vi "I(V)_MFLI_PK_v4.0_measure X.vi"() -> ()   [LabVIEW 2016]
uses:
  Labview Drivers/MFLI/LabOneLabVIEW-22.02.26577/LabOneLabVIEW-22.02.26577/Zurich Instruments LabOne/Public/Data/ziTypeDemodSampleSingle.ctl
  Labview Drivers/MFLI/LabOneLabVIEW-22.02.26577/LabOneLabVIEW-22.02.26577/Zurich Instruments LabOne/Public/Configure/ziSetValueDouble.vi
  Labview Drivers/MFLI/LabOneLabVIEW-22.02.26577/LabOneLabVIEW-22.02.26577/Zurich Instruments LabOne/Public/Configure/ziGetValueDemodSampleEx.vi
  Labview Drivers/MFLI/LabOneLabVIEW-22.02.26577/LabOneLabVIEW-22.02.26577/Zurich Instruments LabOne/Zurich Instruments LabOne.lvlib
panel:
  in  "MFLI Average":i32=1
  out "Resistance (ohm)":dbl=10.271037379735393 format="%#_13g"
  out "R vs V":cluster{dbl, "Field Reading":dbl}[](graph)=[{8.807116465394836e-09, "Field Reading"=-5977.19453137507}, {7.862385412624124e-09, "Field Reading"=0.816626175267259}, {1.016246783678571e-08, "Field Reading"=0.22593081706163012}, {2.8394518144070844e-08, "Field Reading"=0.3244930369790309}, {4.55394808090395e-08, "Field Reading"=0.3437719763523952}, {6.89280912729516e-08, "Field Reading"=0.38589888456590915}, {8.892988920666698e-08, "Field Reading"=0.07130629996454171}, {1.1092974614674399e-07, "Field Reading"=0.2348376343368235}, {1.291523087387538e-07, "Field Reading"=0.37898620517760767}, {1.4722365790221026e-07, "Field Reading"=0.4039183683262634}, {1.807306492808588e-07, "Field Reading"=0.44321715885434587}, {1.9469830782225016e-07, "Field Reading"=0.4299026538647131}, {2.1455394499138842e-07, "Field Reading"=0.43043853663662857}, {2.3655611150765593e-07, "Field Reading"=0.43467611037569903}, {2.59606088721133e-07, "Field Reading"=0.43952372149878877}, {2.758303395650899e-07, "Field Reading"=0.43362275822843394}, {2.898255168785462e-07, "Field Reading"=0.42491475414262025}, {3.1095121503066903e-07, "Field Reading"=0.4281996541380056}, {3.290239859654633e-07, "Field Reading"=0.426217192462996}, {3.440405349336837e-07, "Field Reading"=0.42103190972467763}, {3.67176584323379e-07, "Field Reading"=0.42612243564533486}, {3.8988760409248366e-07, "Field Reading"=0.42973279263530023}, {4.033185654384404e-07, "Field Reading"=0.4229755766582419}, {4.251248472726496e-07, "Field Reading"=0.42533821159897195}, {4.5031688342256917e-07, "Field Reading"=0.43082327628658923}, {4.6749835720727547e-07, "Field Reading"=0.4285130615827359}, {4.868781675265887e-07, "Field Reading"=0.42843576289196017}, {5.115536329406834e-07, "Field Reading"=0.43266001598448733}, {5.343117600631355e-07, "Field Reading"=0.4353606504326838}, {5.541237064759493e-07, "Field Reading"=0.43555248194144336}, {5.726324607401028e-07, "Field Reading"=0.4346915313695261}, {5.873127708721604e-07, "Field Reading"=0.4307903324089991}, {6.019024857908083e-07, "Field Reading"=0.4272258139653861}, {6.223909508091271e-07, "Field Reading"=0.4278930599741731}, {6.425541697267918e-07, "Field Reading"=0.42851691356665206}, {6.687384309745611e-07, "Field Reading"=0.4327338077376769}, {6.88227751334839e-07, "Field Reading"=0.43265173136675905}, {7.032166146053452e-07, "Field Reading"=0.42977933132645724}, {7.224516085197258e-07, "Field Reading"=0.4295413108829304}, {7.474914126034483e-07, "Field Reading"=0.4326650258503734}, {7.733169248070552e-07, "Field Reading"=0.4361152915047444}, {7.885708893571228e-07, "Field Reading"=0.43367432747768353}, {8.069399471456721e-07, "Field Reading"=0.4330162152944697}, {8.337333568827311e-07, "Field Reading"=0.4367253360501215}, {8.502533827097552e-07, "Field Reading"=0.4347849286054917}, {8.646622700555259e-07, "Field Reading"=0.43205649752211134}, {8.808103063521348e-07, "Field Reading"=0.43032588911090636}, {9.07332307666703e-07, "Field Reading"=0.43368905642592026}, {9.20609541766958e-07, "Field Reading"=0.43064678759769065}, {9.413838865796745e-07, "Field Reading"=0.43126579720306557}, {9.58844279524242e-07, "Field Reading"=0.4305551591427947}, {9.970062230902378e-07, "Field Reading"=0.4381510514435691}, {9.96970065778307e-07, "Field Reading"=0.43998698408792436}, {9.807248151559287e-07, "Field Reading"=0.4396609204768114}, {9.60788038185395e-07, "Field Reading"=0.4393338777736508}, {9.372750482786492e-07, "Field Reading"=0.4377520154841891}, {9.195535692551114e-07, "Field Reading"=0.4387479841600016}, {8.938226244658001e-07, "Field Reading"=0.43597257109525617}, {8.749449238095523e-07, "Field Reading"=0.43653094526759}, {8.604976902009871e-07, "Field Reading"=0.43948623716641116}, {8.444380055844986e-07, "Field Reading"=0.44151279280166555}, {8.242449148604546e-07, "Field Reading"=0.4413576911171584}, {8.071962705871049e-07, "Field Reading"=0.44288764318860857}, {7.866878492131972e-07, "Field Reading"=0.4426969475593997}, {7.636574685574939e-07, "Field Reading"=0.4409956934899534}, {7.470356277418868e-07, "Field Reading"=0.4429996029942809}, {7.280251583606455e-07, "Field Reading"=0.4437236899585041}, {7.044622901408893e-07, "Field Reading"=0.44147559373644474}, {6.752061843116512e-07, "Field Reading"=0.4357652741901812}, {6.570212495481336e-07, "Field Reading"=0.43676614696227956}, {6.473149857818308e-07, "Field Reading"=0.44369187060292975}, {6.22864214179742e-07, "Field Reading"=0.4406956990945887}, {6.069148248148923e-07, "Field Reading"=0.44398784538404673}, {5.835665154958818e-07, "Field Reading"=0.4416715102774319}, {5.65865799889914e-07, "Field Reading"=0.4435534098098673}, {5.472677978892445e-07, "Field Reading"=0.4444833144020406}, {5.246199453590136e-07, "Field Reading"=0.4424167859163785}, {5.045265343688379e-07, "Field Reading"=0.4423503207904111}, {4.7659177261486686e-07, "Field Reading"=0.4353927329081167}, {4.5772240158518184e-07, "Field Reading"=0.43594467804068837}, {4.4114317812246226e-07, "Field Reading"=0.439489335160813}, {4.2412032545108266e-07, "Field Reading"=0.44284695573437516}, {4.043466643007711e-07, "Field Reading"=0.44310725253214606}, {3.8417472365546725e-07, "Field Reading"=0.4425432004814173}, {3.7042839611689157e-07, "Field Reading"=0.45040283885873167}, {3.4477591493980703e-07, "Field Reading"=0.4443895189625206}, {3.2725733581528933e-07, "Field Reading"=0.4481410845900496}, {3.081572462473518e-07, "Field Reading"=0.45006110948616496}, {2.8525211285226547e-07, "Field Reading"=0.44584929960121417}, {2.6532424748653286e-07, "Field Reading"=0.44652243638512756}, {2.4966293313200445e-07, "Field Reading"=0.4556278265791199}, {2.2405576218342857e-07, "Field Reading"=0.44610999604451923}, {2.014073596420467e-07, "Field Reading"=0.44110751410180055}, {1.8167493569773264e-07, "Field Reading"=0.44102236093861097}, {1.7140600954601949e-07, "Field Reading"=0.4678237688486504}, {1.5330334235583092e-07, "Field Reading"=0.4776196993681165}, {1.2822346306666566e-07, "Field Reading"=0.4642555634301045}, {1.0593525795964871e-07, "Field Reading"=0.4593885034596967}, {9.055852686825892e-08, "Field Reading"=0.4922634016942269}, {6.797588028856873e-08, "Field Reading"=0.48862602541512123}, {4.555012655190456e-08, "Field Reading"=0.48908283418691806}, {2.9709664516311148e-08, "Field Reading"=0.6129454102917938}, {3.3888522809468195e-10, "Field Reading"=-0.01546163791612826}, {-1.4239079127267004e-08, "Field Reading"=0.28472058806070966}, {-2.8799139958012918e-08, "Field Reading"=0.32155753465506187}, {-4.89750958955916e-08, "Field Reading"=0.36539128711876556}, {-7.520337417178886e-08, "Field Reading"=0.41909212823611885}, {-9.972326582833285e-08, "Field Reading"=0.07997432021548584}, {-1.0990263484124685e-07, "Field Reading"=0.23336629535406556}, {-1.312819662180115e-07, "Field Reading"=0.38487742525414825}, {-1.5592463116991817e-07, "Field Reading"=0.4278153489065379}, {-1.7653875266424058e-07, "Field Reading"=0.4334965056757724}, {-1.971637135376259e-07, "Field Reading"=0.4351792633574556}, {-2.1808458560565266e-07, "Field Reading"=0.4375142673850798}, {-2.3180240935191514e-07, "Field Reading"=0.4264333792769663}, {-2.48554633891114e-07, "Field Reading"=0.42156756387732536}, {-2.6345831908587617e-07, "Field Reading"=0.4147998029873139}, {-2.85570672819698e-07, "Field Reading"=0.4194554633729775}, {-3.1175740482378844e-07, "Field Reading"=0.42978187880042185}, {-3.3278590331955103e-07, "Field Reading"=0.43136965063739224}, {-3.51467501666947e-07, "Field Reading"=0.43012014344692184}, {-3.72178282280472e-07, "Field Reading"=0.4318972800213743}, {-3.9240686597559033e-07, "Field Reading"=0.432121829714655}, {-4.059827115113735e-07, "Field Reading"=0.4253724895675605}, {-4.300880777609571e-07, "Field Reading"=0.4302405035159283}, {-4.504819882312741e-07, "Field Reading"=0.4312258126661519}, {-4.637529480114017e-07, "Field Reading"=0.42550950628327083}, {-4.867159815329638e-07, "Field Reading"=0.42868505140896224}, {-5.077456519616934e-07, "Field Reading"=0.4299220800292077}, {-5.310499523204508e-07, "Field Reading"=0.4328608416660864}, {-5.538076921093847e-07, "Field Reading"=0.43532245858842916}, {-5.702677764394357e-07, "Field Reading"=0.43289823444192205}, {-5.927682391225503e-07, "Field Reading"=0.4347702105544751}, {-6.097202324671173e-07, "Field Reading"=0.4327333005424846}, {-6.296443835385095e-07, "Field Reading"=0.43283028075710905}, {-6.49637385358458e-07, "Field Reading"=0.43321425646099704}, {-6.723806556091608e-07, "Field Reading"=0.43513270916397073}, {-6.884269794808045e-07, "Field Reading"=0.43296467146119394}, {-7.061923905724436e-07, "Field Reading"=0.4315183639881751}, {-7.266464962899468e-07, "Field Reading"=0.4319018109276345}, {-7.424666676907956e-07, "Field Reading"=0.42977521080423625}, {-7.64599974352614e-07, "Field Reading"=0.4313677696204595}, {-7.901898579528715e-07, "Field Reading"=0.434487645528477}, {-8.093035058748168e-07, "Field Reading"=0.43401798183516077}, {-8.20835670236861e-07, "Field Reading"=0.4299052651744387}, {-8.441954463577789e-07, "Field Reading"=0.43193064437269285}, {-8.653366896214197e-07, "Field Reading"=0.43251171114257303}, {-8.865545384944012e-07, "Field Reading"=0.43322530261364495}, {-9.038958737826427e-07, "Field Reading"=0.4323566406327061}, {-9.258281264155032e-07, "Field Reading"=0.43331169068634195}, {-9.467918299486651e-07, "Field Reading"=0.4336274121430956}, {-9.644953806012757e-07, "Field Reading"=0.43272258447089856}, {-1.0060949604233222e-06, "Field Reading"=0.4421351386990255}, {-1.010736976911948e-06, "Field Reading"=0.44609330182465096}, {-9.928102585548402e-07, "Field Reading"=0.44520475124596415}, {-9.766980828813665e-07, "Field Reading"=0.44671425745093024}, {-9.60051969725574e-07, "Field Reading"=0.44820010988159664}, {-9.386970755059166e-07, "Field Reading"=0.44799826313900587}, {-9.201672785553204e-07, "Field Reading"=0.4488492224921183}, {-8.979149299456677e-07, "Field Reading"=0.44787835785073016}, {-8.76460372311859e-07, "Field Reading"=0.44730154712221676}, {-8.530262150140967e-07, "Field Reading"=0.4458907671791061}, {-8.335263634545885e-07, "Field Reading"=0.4463438953650249}, {-8.197783389098899e-07, "Field Reading"=0.4499792105569449}, {-8.038302180821772e-07, "Field Reading"=0.4522995105960239}, {-7.83282457570981e-07, "Field Reading"=0.45222421523328293}, {-7.601831762907309e-07, "Field Reading"=0.4509281744354805}, {-7.389109665306674e-07, "Field Reading"=0.45052666121196844}, {-7.182629250232044e-07, "Field Reading"=0.45030071364752855}, {-7.004340155613462e-07, "Field Reading"=0.4517544079032464}, {-6.814395854673362e-07, "Field Reading"=0.4529276191992989}, {-6.558300686969053e-07, "Field Reading"=0.4493277209727905}, {-6.359316180937803e-07, "Field Reading"=0.4500290849336199}, {-6.154748982876061e-07, "Field Reading"=0.45020306366458507}, {-5.917094945813965e-07, "Field Reading"=0.44789414822583756}, {-5.73965480045129e-07, "Field Reading"=0.4497842743714328}, {-5.545982163184653e-07, "Field Reading"=0.4504797232919903}, {-5.351247253506258e-07, "Field Reading"=0.45088817354744287}, {-5.152527552615877e-07, "Field Reading"=0.4520701157056494}, {-5.006045613860368e-07, "Field Reading"=0.45775214570075445}, {-4.780418528862968e-07, "Field Reading"=0.45561649417384475}, {-4.548773141292071e-07, "Field Reading"=0.4532294398774025}, {-4.357141013306226e-07, "Field Reading"=0.45497073363885965}, {-4.207081751843158e-07, "Field Reading"=0.4615871705693569}, {-3.922877082311092e-07, "Field Reading"=0.4525844537936392}, {-3.692015436639742e-07, "Field Reading"=0.4493167461190504}, {-3.509956335404888e-07, "Field Reading"=0.45168466588578915}, {-3.360460006702773e-07, "Field Reading"=0.46029053735098013}, {-3.1020545935161133e-07, "Field Reading"=0.45316592355628316}, {-2.8989555441284607e-07, "Field Reading"=0.45333098233399943}, {-2.669248728421333e-07, "Field Reading"=0.44909538161604934}, {-2.489744492703013e-07, "Field Reading"=0.4533128411658068}, {-2.2787063234470874e-07, "Field Reading"=0.45336736758430596}, {-2.0728620353717052e-07, "Field Reading"=0.45370367315504495}, {-1.884405207301443e-07, "Field Reading"=0.4576065563919088}, {-1.635396043180527e-07, "Field Reading"=0.4448754526645907}, {-1.4583051153218797e-07, "Field Reading"=0.4551764116154708}, {-1.242145557742591e-07, "Field Reading"=0.45282925083043807}, {-1.0703780792300653e-07, "Field Reading"=0.46739265389657464}, {-8.94525755579511e-08, "Field Reading"=0.48614795183788406}, {-6.707150413797107e-08, "Field Reading"=0.4822484375591752}, {-5.213931166691103e-08, "Field Reading"=0.5613075844182088}, {-2.742894167784647e-08, "Field Reading"=10.271037379735393}]
  out "Set Voltage(V)":dbl=-1.452335524282492e-15 format="%#_13g"
  out "Time(s)":dbl=2806.269 format="%#_13g"
  out "Demod Sample Out 2":T1={"Timestamps (ticks)"=512980697382069, "X (Vrms)"=-2.0613062921871483e-09, "Y (Vrms)"=4.065821120622337e-09, "Osc Phase (deg)"=5.281591726489506, "Freq (Hz)"=3.998000011051772, "DIO"=0, "AuxIn0 (V)"=0.0, "AuxIn1 (V)"=0.0003350508341100067, "Trigger"=768}
  out "Demod Sample Out":T1={"Timestamps (ticks)"=512980637206709, "X (Vrms)"=-2.4994520688007507e-08, "Y (Vrms)"=1.0539359089071451e-08, "Osc Phase (deg)"=4.127175309806318, "Freq (Hz)"=3.998000011051772, "DIO"=0, "AuxIn0 (V)"=-0.0010006982192862779, "AuxIn1 (V)"=0.0026804066728800535, "Trigger"=768}
  in  "MFLI Current source/Voltage reader":string="DEV3647"
  out "Imeas (A)":dbl=-2.6705132757050783e-09
  out "Vmeas (V)":dbl=-2.742894167784647e-08
  in  "Folder":path=path "D:/Banabir/sixth_round/10-11-2021"
  in  "wait (ms) [Should be > TC]":u32=1000
  out "I vs V":cluster{dbl, "Field Reading":dbl}[](graph)=[{8.807116465394836e-09, "Field Reading"=-1.4734532093886417e-12}, {7.862385412624124e-09, "Field Reading"=9.62788807259452e-09}, {1.016246783678571e-08, "Field Reading"=4.498044122070147e-08}, {2.8394518144070844e-08, "Field Reading"=8.750424480111642e-08}, {4.55394808090395e-08, "Field Reading"=1.32470020657989e-07}, {6.89280912729516e-08, "Field Reading"=1.7861697462662426e-07}, {8.892988920666698e-08, "Field Reading"=1.247153326576879e-06}, {1.1092974614674399e-07, "Field Reading"=4.723678402740142e-07}, {1.291523087387538e-07, "Field Reading"=3.4078366698921936e-07}, {1.4722365790221026e-07, "Field Reading"=3.644886428717472e-07}, {1.807306492808588e-07, "Field Reading"=4.077699738611703e-07}, {1.9469830782225016e-07, "Field Reading"=4.5288929033576084e-07}, {2.1455394499138842e-07, "Field Reading"=4.984543128221637e-07}, {2.3655611150765593e-07, "Field Reading"=5.442123591820951e-07}, {2.59606088721133e-07, "Field Reading"=5.906531912222363e-07}, {2.758303395650899e-07, "Field Reading"=6.361066948884209e-07}, {2.898255168785462e-07, "Field Reading"=6.820792030706185e-07}, {3.1095121503066903e-07, "Field Reading"=7.261827795182005e-07}, {3.290239859654633e-07, "Field Reading"=7.719631957221647e-07}, {3.440405349336837e-07, "Field Reading"=8.171364853525227e-07}, {3.67176584323379e-07, "Field Reading"=8.616692143123462e-07}, {3.8988760409248366e-07, "Field Reading"=9.072791529395062e-07}, {4.033185654384404e-07, "Field Reading"=9.535268410173856e-07}, {4.251248472726496e-07, "Field Reading"=9.994983654877368e-07}, {4.5031688342256917e-07, "Field Reading"=1.0452473397073666e-06}, {4.6749835720727547e-07, "Field Reading"=1.0909780800625897e-06}, {4.868781675265887e-07, "Field Reading"=1.1364087914606841e-06}, {5.115536329406834e-07, "Field Reading"=1.1823455231394082e-06}, {5.343117600631355e-07, "Field Reading"=1.227285377151355e-06}, {5.541237064759493e-07, "Field Reading"=1.2722317733238103e-06}, {5.726324607401028e-07, "Field Reading"=1.3173306112865464e-06}, {5.873127708721604e-07, "Field Reading"=1.3633378622678943e-06}, {6.019024857908083e-07, "Field Reading"=1.4088626345026393e-06}, {6.223909508091271e-07, "Field Reading"=1.45454789766091e-06}, {6.425541697267918e-07, "Field Reading"=1.4994837995510021e-06}, {6.687384309745611e-07, "Field Reading"=1.5453805989199487e-06}, {6.88227751334839e-07, "Field Reading"=1.5907199750725789e-06}, {7.032166146053452e-07, "Field Reading"=1.6362271597262713e-06}, {7.224516085197258e-07, "Field Reading"=1.6819141493858012e-06}, {7.474914126034483e-07, "Field Reading"=1.7276446394859515e-06}, {7.733169248070552e-07, "Field Reading"=1.77319378584239e-06}, {7.885708893571228e-07, "Field Reading"=1.8183480999292075e-06}, {8.069399471456721e-07, "Field Reading"=1.8635328623823433e-06}, {8.337333568827311e-07, "Field Reading"=1.9090565352202197e-06}, {8.502533827097552e-07, "Field Reading"=1.9555723457039254e-06}, {8.646622700555259e-07, "Field Reading"=2.001271303670824e-06}, {8.808103063521348e-07, "Field Reading"=2.046844795166685e-06}, {9.07332307666703e-07, "Field Reading"=2.0921263615552797e-06}, {9.20609541766958e-07, "Field Reading"=2.137736930310019e-06}, {9.413838865796745e-07, "Field Reading"=2.18283919727679e-06}, {9.58844279524242e-07, "Field Reading"=2.226995215742471e-06}, {9.970062230902378e-07, "Field Reading"=2.275485177555589e-06}, {9.96970065778307e-07, "Field Reading"=2.2659080878153395e-06}, {9.807248151559287e-07, "Field Reading"=2.23063904358917e-06}, {9.60788038185395e-07, "Field Reading"=2.1869199868087628e-06}, {9.372750482786492e-07, "Field Reading"=2.1411096125781333e-06}, {9.195535692551114e-07, "Field Reading"=2.095858220330354e-06}, {8.938226244658001e-07, "Field Reading"=2.050180868535667e-06}, {8.749449238095523e-07, "Field Reading"=2.004313630671058e-06}, {8.604976902009871e-07, "Field Reading"=1.9579627697764748e-06}, {8.444380055844986e-07, "Field Reading"=1.9126014451948923e-06}, {8.242449148604546e-07, "Field Reading"=1.8675213584114449e-06}, {8.071962705871049e-07, "Field Reading"=1.8225757322458227e-06}, {7.866878492131972e-07, "Field Reading"=1.777034726691089e-06}, {7.636574685574939e-07, "Field Reading"=1.731666498858659e-06}, {7.470356277418868e-07, "Field Reading"=1.6863121833351416e-06}, {7.280251583606455e-07, "Field Reading"=1.6407173536953336e-06}, {7.044622901408893e-07, "Field Reading"=1.5956992869722358e-06}, {6.752061843116512e-07, "Field Reading"=1.549472214293447e-06}, {6.570212495481336e-07, "Field Reading"=1.504286113101334e-06}, {6.473149857818308e-07, "Field Reading"=1.4589291097495182e-06}, {6.22864214179742e-07, "Field Reading"=1.4133657656732736e-06}, {6.069148248148923e-07, "Field Reading"=1.3669627020755822e-06}, {5.835665154958818e-07, "Field Reading"=1.3212681866877033e-06}, {5.65865799889914e-07, "Field Reading"=1.275755720449713e-06}, {5.472677978892445e-07, "Field Reading"=1.2312448637705984e-06}, {5.246199453590136e-07, "Field Reading"=1.1858047932615566e-06}, {5.045265343688379e-07, "Field Reading"=1.1405587622663585e-06}, {4.7659177261486686e-07, "Field Reading"=1.0946250054096438e-06}, {4.5772240158518184e-07, "Field Reading"=1.0499552457948825e-06}, {4.4114317812246226e-07, "Field Reading"=1.0037631014664874e-06}, {4.2412032545108266e-07, "Field Reading"=9.577130879171608e-07}, {4.043466643007711e-07, "Field Reading"=9.125254935235731e-07}, {3.8417472365546725e-07, "Field Reading"=8.681067141864243e-07}, {3.7042839611689157e-07, "Field Reading"=8.224379692088842e-07}, {3.4477591493980703e-07, "Field Reading"=7.758416889415547e-07}, {3.2725733581528933e-07, "Field Reading"=7.302551519342569e-07}, {3.081572462473518e-07, "Field Reading"=6.84700898949423e-07}, {2.8525211285226547e-07, "Field Reading"=6.397949107633602e-07}, {2.6532424748653286e-07, "Field Reading"=5.942013790717776e-07}, {2.4966293313200445e-07, "Field Reading"=5.479536555229478e-07}, {2.2405576218342857e-07, "Field Reading"=5.022433125687439e-07}, {2.014073596420467e-07, "Field Reading"=4.565947149011048e-07}, {1.8167493569773264e-07, "Field Reading"=4.119404179667463e-07}, {1.7140600954601949e-07, "Field Reading"=3.663901258541493e-07}, {1.5330334235583092e-07, "Field Reading"=3.209736586632605e-07}, {1.2822346306666566e-07, "Field Reading"=2.7619154872221623e-07}, {1.0593525795964871e-07, "Field Reading"=2.3060058569563808e-07}, {9.055852686825892e-08, "Field Reading"=1.839635580394214e-07}, {6.797588028856873e-08, "Field Reading"=1.391163727532085e-07}, {4.555012655190456e-08, "Field Reading"=9.313376665044878e-08}, {2.9709664516311148e-08, "Field Reading"=4.8470327075567474e-08}, {3.3888522809468195e-10, "Field Reading"=-2.191780909195822e-08}, {-1.4239079127267004e-08, "Field Reading"=-5.0010711288046624e-08}, {-2.8799139958012918e-08, "Field Reading"=-8.956139058879792e-08}, {-4.89750958955916e-08, "Field Reading"=-1.3403465715282067e-07}, {-7.520337417178886e-08, "Field Reading"=-1.7944353784048852e-07}, {-9.972326582833285e-08, "Field Reading"=-1.2469410875845484e-06}, {-1.0990263484124685e-07, "Field Reading"=-4.7094476378648224e-07}, {-1.312819662180115e-07, "Field Reading"=-3.4110071831654284e-07}, {-1.5592463116991817e-07, "Field Reading"=-3.644671271576608e-07}, {-1.7653875266424058e-07, "Field Reading"=-4.072437732549573e-07}, {-1.971637135376259e-07, "Field Reading"=-4.530632089784938e-07}, {-2.1808458560565266e-07, "Field Reading"=-4.984627973599423e-07}, {-2.3180240935191514e-07, "Field Reading"=-5.435841109458757e-07}, {-2.48554633891114e-07, "Field Reading"=-5.89596200440702e-07}, {-2.6345831908587617e-07, "Field Reading"=-6.351457189432023e-07}, {-2.85570672819698e-07, "Field Reading"=-6.80812857992912e-07}, {-3.1175740482378844e-07, "Field Reading"=-7.25385178393153e-07}, {-3.3278590331955103e-07, "Field Reading"=-7.714634138674945e-07}, {-3.51467501666947e-07, "Field Reading"=-8.171379718474384e-07}, {-3.72178282280472e-07, "Field Reading"=-8.617287014682129e-07}, {-3.9240686597559033e-07, "Field Reading"=-9.080931325193873e-07}, {-4.059827115113735e-07, "Field Reading"=-9.544169438980435e-07}, {-4.300880777609571e-07, "Field Reading"=-9.99645719652786e-07}, {-4.504819882312741e-07, "Field Reading"=-1.0446545058285506e-06}, {-4.637529480114017e-07, "Field Reading"=-1.0898768209955605e-06}, {-4.867159815329638e-07, "Field Reading"=-1.1353696144366847e-06}, {-5.077456519616934e-07, "Field Reading"=-1.181017853112356e-06}, {-5.310499523204508e-07, "Field Reading"=-1.2268375912139185e-06}, {-5.538076921093847e-07, "Field Reading"=-1.272178085884092e-06}, {-5.702677764394357e-07, "Field Reading"=-1.3173252535312505e-06}, {-5.927682391225503e-07, "Field Reading"=-1.363405828487135e-06}, {-6.097202324671173e-07, "Field Reading"=-1.4089977168448967e-06}, {-6.296443835385095e-07, "Field Reading"=-1.4547142645314281e-06}, {-6.49637385358458e-07, "Field Reading"=-1.4995752694416368e-06}, {-6.723806556091608e-07, "Field Reading"=-1.5452312396855188e-06}, {-6.884269794808045e-07, "Field Reading"=-1.5900303762832697e-06}, {-7.061923905724436e-07, "Field Reading"=-1.6365291711937327e-06}, {-7.266464962899468e-07, "Field Reading"=-1.6824344744683115e-06}, {-7.424666676907956e-07, "Field Reading"=-1.7275697830533812e-06}, {-7.64599974352614e-07, "Field Reading"=-1.7725013971844722e-06}, {-7.901898579528715e-07, "Field Reading"=-1.8186704871475597e-06}, {-8.093035058748168e-07, "Field Reading"=-1.864677363027297e-06}, {-8.20835670236861e-07, "Field Reading"=-1.90934081699092e-06}, {-8.441954463577789e-07, "Field Reading"=-1.9544699070468404e-06}, {-8.653366896214197e-07, "Field Reading"=-2.0007242979281327e-06}, {-8.865545384944012e-07, "Field Reading"=-2.046405261063526e-06}, {-9.038958737826427e-07, "Field Reading"=-2.090625629017496e-06}, {-9.258281264155032e-07, "Field Reading"=-2.1366331587985596e-06}, {-9.467918299486651e-07, "Field Reading"=-2.183422457702529e-06}, {-9.644953806012757e-07, "Field Reading"=-2.2289000279026107e-06}, {-1.0060949604233222e-06, "Field Reading"=-2.275537211052119e-06}, {-1.010736976911948e-06, "Field Reading"=-2.265752417213486e-06}, {-9.928102585548402e-07, "Field Reading"=-2.2300082282956997e-06}, {-9.766980828813665e-07, "Field Reading"=-2.186404545166443e-06}, {-9.60051969725574e-07, "Field Reading"=-2.1420163640281033e-06}, {-9.386970755059166e-07, "Field Reading"=-2.095314095480445e-06}, {-9.201672785553204e-07, "Field Reading"=-2.0500587556915694e-06}, {-8.979149299456677e-07, "Field Reading"=-2.0048187509094304e-06}, {-8.76460372311859e-07, "Field Reading"=-1.959439617302246e-06}, {-8.530262150140967e-07, "Field Reading"=-1.9130833778207653e-06}, {-8.335263634545885e-07, "Field Reading"=-1.8674532621823393e-06}, {-8.197783389098899e-07, "Field Reading"=-1.8218138075651095e-06}, {-8.038302180821772e-07, "Field Reading"=-1.7772077998114984e-06}, {-7.83282457570981e-07, "Field Reading"=-1.7320665970240434e-06}, {-7.601831762907309e-07, "Field Reading"=-1.6858187609199812e-06}, {-7.389109665306674e-07, "Field Reading"=-1.6401048598165359e-06}, {-7.182629250232044e-07, "Field Reading"=-1.5950739211695374e-06}, {-7.004340155613462e-07, "Field Reading"=-1.5504752212874042e-06}, {-6.814395854673362e-07, "Field Reading"=-1.5045220396848587e-06}, {-6.558300686969053e-07, "Field Reading"=-1.459580698197385e-06}, {-6.359316180937803e-07, "Field Reading"=-1.4130900410305286e-06}, {-6.154748982876061e-07, "Field Reading"=-1.3671050864863805e-06}, {-5.917094945813965e-07, "Field Reading"=-1.3210922646014216e-06}, {-5.73965480045129e-07, "Field Reading"=-1.2760905899772456e-06}, {-5.545982163184653e-07, "Field Reading"=-1.2311280344997632e-06}, {-5.351247253506258e-07, "Field Reading"=-1.1868236000523963e-06}, {-5.152527552615877e-07, "Field Reading"=-1.139762920310082e-06}, {-5.006045613860368e-07, "Field Reading"=-1.0936148876368046e-06}, {-4.780418528862968e-07, "Field Reading"=-1.0492198131525403e-06}, {-4.548773141292071e-07, "Field Reading"=-1.0036358499841722e-06}, {-4.357141013306226e-07, "Field Reading"=-9.576750087764496e-07}, {-4.207081751843158e-07, "Field Reading"=-9.114381898122996e-07}, {-3.922877082311092e-07, "Field Reading"=-8.667723889826252e-07}, {-3.692015436639742e-07, "Field Reading"=-8.216954895470354e-07}, {-3.509956335404888e-07, "Field Reading"=-7.770811365760198e-07}, {-3.360460006702773e-07, "Field Reading"=-7.300736673933315e-07}, {-3.1020545935161133e-07, "Field Reading"=-6.84529535930748e-07}, {-2.8989555441284607e-07, "Field Reading"=-6.39478804030342e-07}, {-2.669248728421333e-07, "Field Reading"=-5.943612064804948e-07}, {-2.489744492703013e-07, "Field Reading"=-5.492331711362986e-07}, {-2.2787063234470874e-07, "Field Reading"=-5.026180723127036e-07}, {-2.0728620353717052e-07, "Field Reading"=-4.5687574468089936e-07}, {-1.884405207301443e-07, "Field Reading"=-4.117959371385358e-07}, {-1.635396043180527e-07, "Field Reading"=-3.6760761543153e-07}, {-1.4583051153218797e-07, "Field Reading"=-3.203824007808743e-07}, {-1.242145557742591e-07, "Field Reading"=-2.743077121154686e-07}, {-1.0703780792300653e-07, "Field Reading"=-2.2901046268196594e-07}, {-8.94525755579511e-08, "Field Reading"=-1.840027819098596e-07}, {-6.707150413797107e-08, "Field Reading"=-1.3908081170245562e-07}, {-5.213931166691103e-08, "Field Reading"=-9.288902041285091e-08}, {-2.742894167784647e-08, "Field Reading"=-2.6705132757050783e-09}]
  out "data":dbl[](array[numeric])=[-2.742894167784647e-08, -2.6705132757050783e-09, 10.271037379735393, -1.0269562977782698e-15, 2806.269]
  in  "Step":dbl[](array[numeric])=[0.1, 0.1, 0.1] min=-3000.0 max=3000.0 format="%.1e"
  in  "To":dbl[](array[numeric])=[5.0, -5.0, 0.0] min=-3000.0 max=3000.0 format="%.1e"
  in  "From":dbl[](array[numeric])=[0.0, 5.0, -5.0] min=-3000.0 max=3000.0 format="%.1e"
  in  "file name":string="004_NTJJ01_450nm_AC_IV_I_98_V_45_14K_0deg(Yaxis)_3.998Hz_1s_1ave_20mT"
  out "File path":path=path "D:/Banabir/sixth_round/10-11-2021/003_NTJJ01_450nm_AC_IV_I_98_V_45_14K_0deg(Yaxis)_3.998Hz_1s_20ave_ZF.dat"
  # ".dat"
  # "Set MFLI Voltage output (V)"
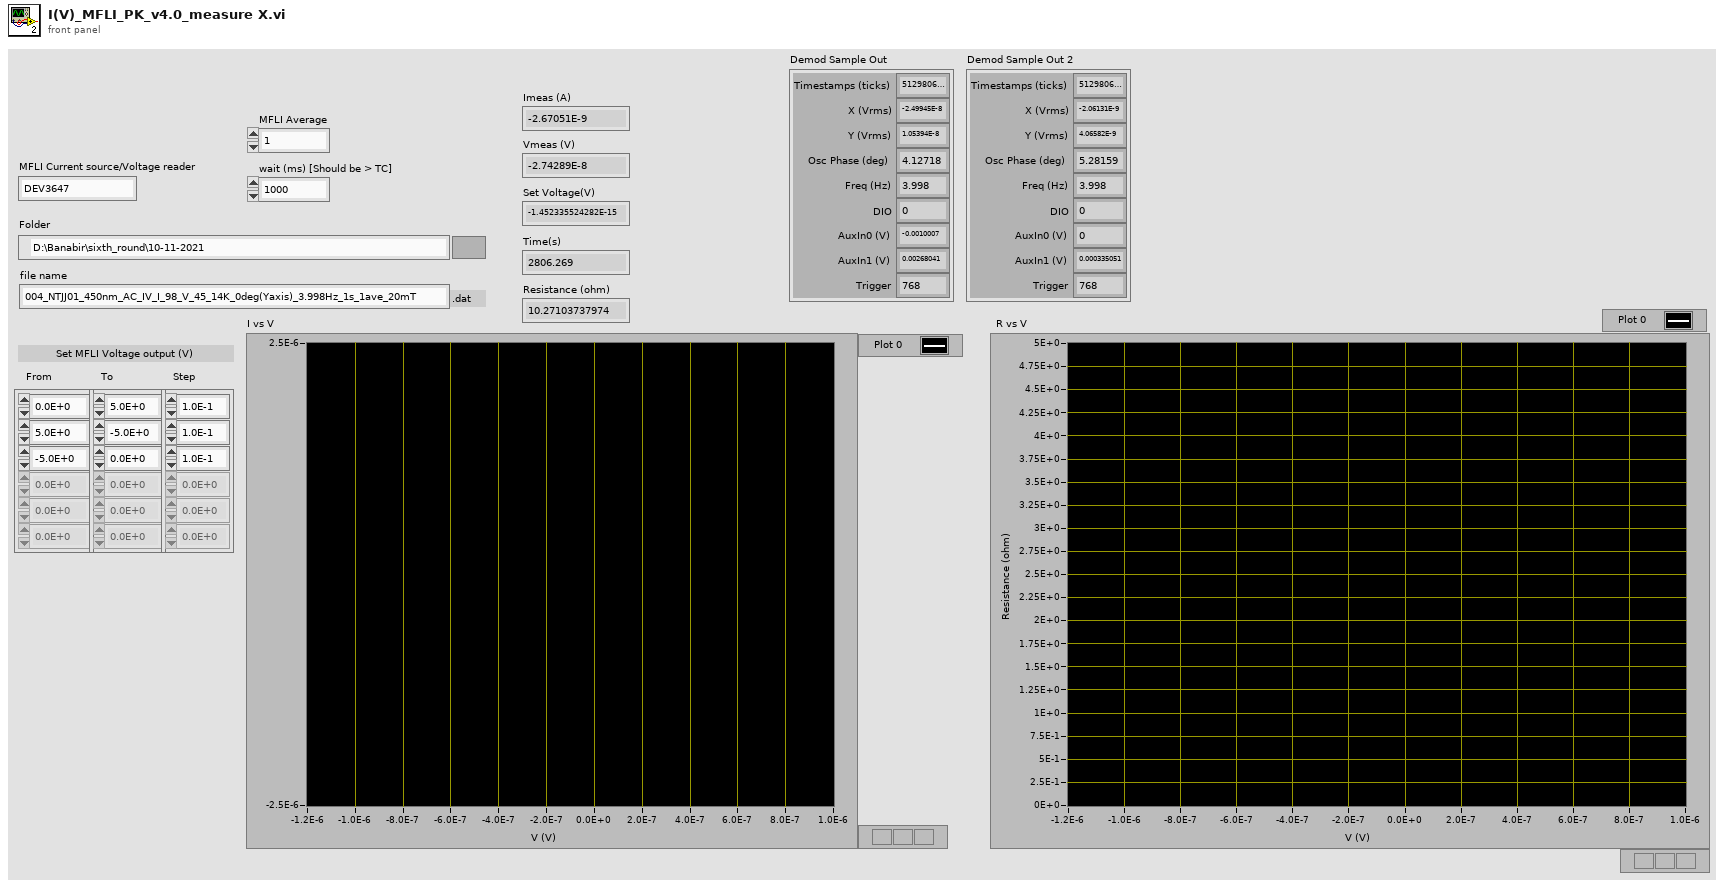
[diagram p1: front panel]
types:
  T1 = typedef "Zurich Instruments LabOne.lvlib/ziTypeDemodSampleSingle.ctl" = cluster{"Timestamps (ticks)":u64, "X (Vrms)":dbl, "Y (Vrms)":dbl, "Osc Phase (deg)":dbl, "Freq (Hz)":dbl, "DIO":u32, "AuxIn0 (V)":dbl, "AuxIn1 (V)":dbl, "Trigger":u32}
  T2 = enum16{"open", "replace", "create", "open or create", "replace or create", "replace or create with confirmation"}
  T3 = typedef "Zurich Instruments LabOne.lvlib/ziTypeHandle.ctl" = cluster{"handleValid":bool, "Conn":u64, "Path Prefix":string, "Handle":u64, "Connected":bool, "Clockbase(s)":dbl}
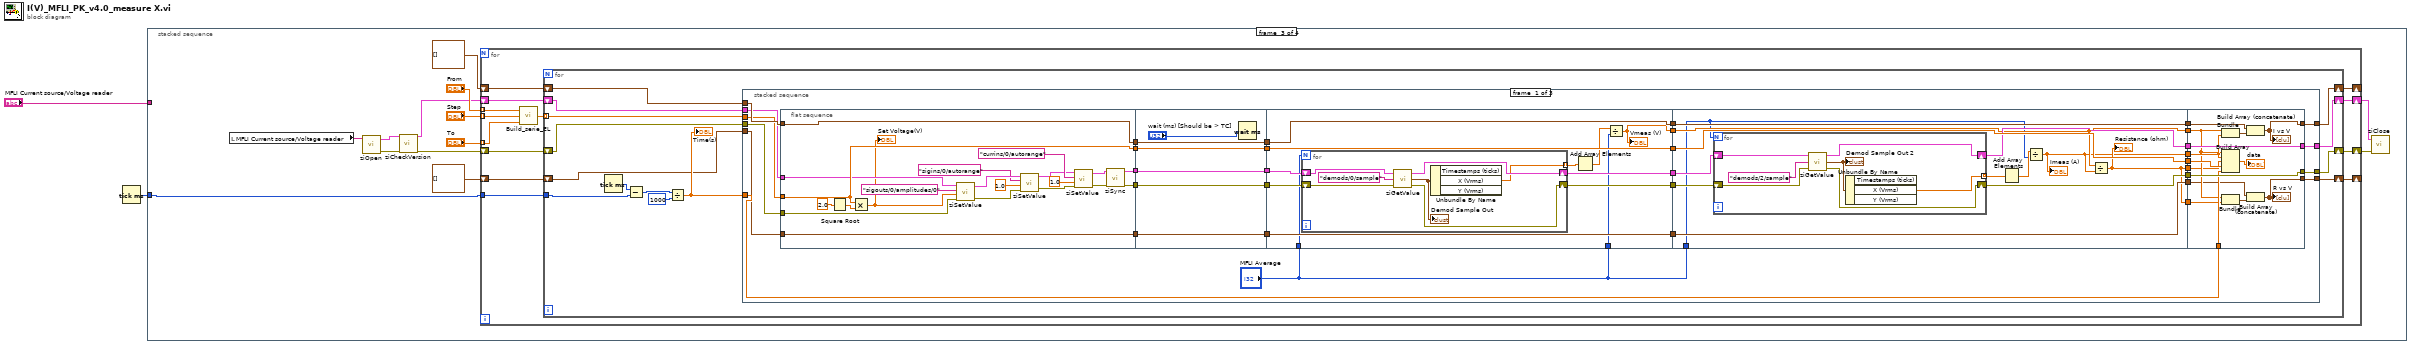
[diagram p0: block diagram]
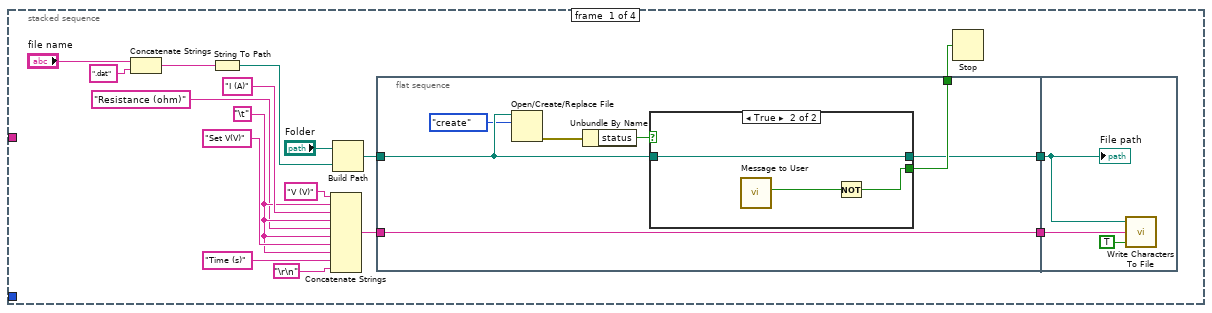
[diagram p2: hidden frame]
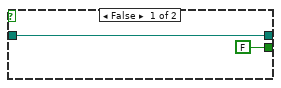
[diagram p3: hidden frame]
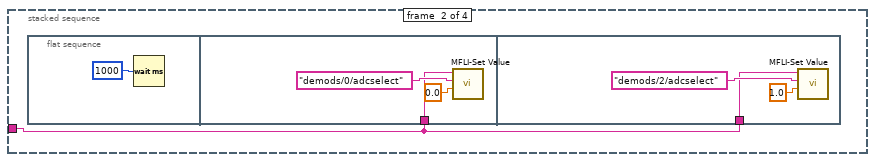
[diagram p4: hidden frame]
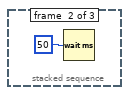
[diagram p5: hidden frame]
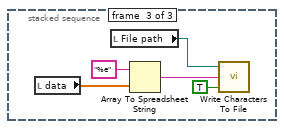
[diagram p6: hidden frame]
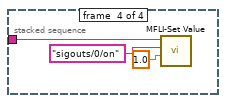
[diagram p7: hidden frame]
diagram:
  n1 = Tick Count (ms)() -> (millisecond timer value=w1:u32)
  n2 = stacked-sequence {
    tunnel: "MFLI Current source/Voltage reader" -> [_ w35 _ w206]
    tunnel: w1 -> [_ _ w51 _]
    frame #0 {
      w4 = "\t"
      n3 = Concatenate Strings("file name", ".dat" ("string")) -> (w16:string)
      n4 = String To Path(string=w16) -> (path=w8:path)
      n5 = Concatenate Strings("V (V)" ("string"), w4, "I (A)" ("string"), w4, "Resistance (ohm)", w4, "Set V(V)" ("string"), w4, "Time (s)", "\r\n") -> (w17:string)
      n6 = Build Path(base path="Folder", name or relative path=w8) -> (appended path=w7:path)
      n7 = flat-sequence {
        tunnel: w7 -> [w23]
        tunnel: w17 -> [w26]
        tunnel: [w26] -> w19
        tunnel: [w25] -> w14
        tunnel: [w24] -> w18
        tunnel: w19 -> [w33]
        tunnel: w18 -> [w32]
        frame #0 {
          n8 = Open/Create/Replace File(file path (use dialog)=w23, operation (0:open)=T2."create") -> (error out=w22:errorcluster)  [unwired: 4 in, 2 out]
          n9 = Unbundle By Name(w22) -> ("status"=w20:bool)
          n10 = case shown="True" w20 {
            tunnel: [FALSE ("Yes") w30] -> w25
            tunnel: [w27 w29] -> w24
            tunnel: w23 -> [w27 w29]
            frame False {
            }
            frame True {
              n11 = call "Message to User"() -> ("Yes"=w31:bool)  [unwired: 10 in, 1 out]
              n12 = Not(x=w31) -> (.not. x?=w30:bool)
            }
          }
        }
        frame #1 {
          n13 = call <vilib>:"Write Characters To File.vi"("append to file? (new file:F)"=TRUE, "character string"=w33, "file path (dialog if empty)"=w32) -> ()  [unwired: 2 in, 1 out]
          "File path" <- w32
        }
      }
      n14 = Stop(stop? (T)=w14) -> ()
    }
    frame #1 {
      n15 = flat-sequence {
        tunnel: w35 -> [w37]
        tunnel: w35 -> [w40]
        frame #0 {
          n16 = Wait (ms)(milliseconds to wait=u32 1000) -> ()  [unwired: 1 out]
        }
        frame #1 {
          n17 = call "MFLI-Set Value.vi"("Value"=0.0, "Path"="demods/0/adcselect", "MFLI Current source/Voltage reader"=w37) -> ()  [unwired: 9 in]
        }
        frame #2 {
          n18 = call "MFLI-Set Value.vi"("Value"=1.0, "Path"="demods/2/adcselect", "MFLI Current source/Voltage reader"=w40) -> ()  [unwired: 9 in]
        }
      }
    }
    frame #2 {
      n19 = local read "MFLI Current source/Voltage reader"() -> (w47:string)
      n20 = call "ziOpen.vi"("Address"=w47) -> ("Error Out"=w48:errorcluster, "HandleOut"=w49:T3)  [unwired: 3 in, 1 out]
      n21 = call "ziCheckVersion.vi"("Handle In"=w49, "Error In"=w48) -> ("Handle Out"=w46:T3, "Error Out"=w45:errorcluster)  [unwired: 11 in, 1 out]
      n22 = for {
        tunnel: "From" -> [w65] mode=indexing
        tunnel: "To" -> [w64] mode=indexing
        tunnel: "Step" -> [w63] mode=indexing
        shift-right: [w67] -> _
        shift-left: cluster{dbl, "Field Reading":dbl}[] [] -> [w68]
        tunnel: w51 -> [w62]
        shift-right: [w61] -> _
        shift-left: cluster{dbl, "Field Reading":dbl}[] [] -> [w60]
        shift-right: [w57] -> w44
        shift-left: w46 -> [w59]
        shift-right: [w56] -> w43
        shift-left: w45 -> [w58]
        n23 = call "Build_serie_EL.vi"("end value"=w64, "increment"=w63, "start value"=w65) -> ("output array"=w66:dbl[])
        n24 = for {
          tunnel: w66 -> [w82] mode=indexing
          shift-right: [w80] -> w67
          shift-left: w68 -> [w81]
          shift-right: [w77] -> w57
          shift-left: w59 -> [w79]
          shift-right: [w76] -> w56
          shift-left: w58 -> [w78]
          tunnel: w62 -> [w72]
          shift-right: [w70] -> w61
          shift-left: w60 -> [w69]
          n25 = Tick Count (ms)() -> (millisecond timer value=w73:u32)
          n26 = Subtract(x=w73, y=w72) -> (x-y=w74:u32)
          n27 = Divide(x=w74, y=1000) -> (x/y=w71:dbl)
          "Time(s)" <- w71
          n28 = stacked-sequence {
            tunnel: w82 -> [w116 _ _]
            tunnel: w81 -> [w117 _ _]
            tunnel: [w118 _ _] -> w80
            tunnel: w79 -> [w107 _ _]
            tunnel: w78 -> [w106 _ _]
            tunnel: [w96 _ _] -> w77
            tunnel: [w95 _ _] -> w76
            tunnel: w71 -> [w92 _ _]
            tunnel: [w90 _ _] -> w70
            tunnel: w69 -> [w85 _ _]
            frame #0 {
              n29 = flat-sequence {
                tunnel: [w139] -> w113
                tunnel: [w138] -> w112
                tunnel: w116 -> [w138]
                tunnel: w117 -> [w139]
                tunnel: [w121] -> w109
                tunnel: [w122] -> w108
                tunnel: w107 -> [w124]
                tunnel: w106 -> [w123]
                tunnel: w85 -> [w119]
                tunnel: [w119] -> w89
                tunnel: w113 -> [w145]
                tunnel: [w145] -> w115
                tunnel: w112 -> [w144]
                tunnel: [w144] -> w114
                tunnel: [w142] -> w111
                tunnel: [w141] -> w110
                tunnel: w109 -> [w141]
                tunnel: w108 -> [w142]
                tunnel: w89 -> [w140]
                tunnel: [w140] -> w88
                tunnel: [w147] -> w105
                tunnel: [w157] -> w103
                tunnel: [w156] -> w101
                tunnel: w110 -> [w155]
                tunnel: w111 -> [w154]
                tunnel: w115 -> [w157]
                tunnel: w114 -> [w156]
                tunnel: [w153] -> w99
                tunnel: [w152] -> w98
                tunnel: w88 -> [w151]
                tunnel: [w151] -> w87
                tunnel: "MFLI Average" -> [w148]
                tunnel: "MFLI Average" -> [w146]
                tunnel: w105 -> [w171]
                tunnel: [w171] -> w104
                tunnel: w103 -> [w177]
                tunnel: [w177] -> w102
                tunnel: w101 -> [w176]
                tunnel: [w176] -> w100
                tunnel: w99 -> [w175]
                tunnel: w98 -> [w174]
                tunnel: [w173] -> w97
                tunnel: [w172] -> w94
                tunnel: [w166] -> w93
                tunnel: [w169] -> w91
                tunnel: w87 -> [w170]
                tunnel: [w170] -> w86
                tunnel: [w169] -> w84
                tunnel: "MFLI Average" -> [w165]
                tunnel: w104 -> [w189]
                tunnel: [w198] -> w118
                tunnel: w102 -> [w197]
                tunnel: w100 -> [w196]
                tunnel: [w195] -> w96
                tunnel: w97 -> [w195]
                tunnel: [w194] -> w95
                tunnel: w94 -> [w194]
                tunnel: w93 -> [w193]
                tunnel: w92 -> [w191]
                tunnel: w91 -> [w188]
                tunnel: [w187] -> w90
                tunnel: w86 -> [w186]
                tunnel: w84 -> [w185]
                frame #0 {
                  n30 = Square Root(x=2.0) -> (sqrt(x)=w137:dbl)
                  n31 = Multiply(x=w138, y=w137) -> (x*y=w120:dbl)
                  "Set Voltage(V)" <- w120
                  n32 = call-poly "ziSetValue.vi"("Error In"=w123, "Value"=w120, "Path"="sigouts/0/amplitudes/0", "Handle In"=w124) -> ("Error Out"=w131:errorcluster, "Handle Out"=w134:T3)  [unwired: 1 in]
                  n33 = call-poly "ziSetValue.vi"("Error In"=w131, "Value"=1.0, "Path"="sigins/0/autorange", "Handle In"=w134) -> ("Error Out"=w127:errorcluster, "Handle Out"=w128:T3)  [unwired: 1 in]
                  n34 = call-poly "ziSetValue.vi"("Error In"=w127, "Value"=1.0, "Path"="currins/0/autorange", "Handle In"=w128) -> ("Error Out"=w125:errorcluster, "Handle Out"=w126:T3)  [unwired: 1 in]
                  n35 = call "ziSync.vi"("Handle In"=w126, "Error In"=w125) -> ("Handle Out"=w122:T3, "Error Out"=w121:errorcluster)  [unwired: 12 in]
                }
                frame #1 {
                  n36 = Wait (ms)(milliseconds to wait="wait (ms) [Should be > TC]") -> ()  [unwired: 1 out]
                }
                frame #2 {
                  n37 = for {
                    N: w146 -> [_]
                    tunnel: [w158] -> w150 mode=indexing
                    shift-right: [w159] -> w152
                    shift-left: w155 -> [w162]
                    shift-right: [w160] -> w153
                    shift-left: w154 -> [w161]
                    n38 = call-poly "ziGetValue.vi"("error in"=w162, "Path"="demods/0/sample", "Handle In"=w161) -> ("error out"=w159:errorcluster, "Demod Sample Out"=w163:T1, "Handle Out"=w160:T3)
                    "Demod Sample Out" <- w163
                    n39 = Unbundle By Name(w163) -> ("X (Vrms)"=w158:dbl)  [unwired: 2 out]
                  }
                  n40 = Add Array Elements(numeric array=w150) -> (sum=w149:dbl)
                  n41 = Divide(x=w149, y=w148) -> (x/y=w147:dbl)
                  "Vmeas (V)" <- w147
                }
                frame #3 {
                  n42 = for {
                    N: w165 -> [_]
                    tunnel: [w178] -> w168 mode=indexing
                    shift-right: [w180] -> w173
                    shift-left: w175 -> [w182]
                    shift-right: [w179] -> w172
                    shift-left: w174 -> [w181]
                    n43 = call-poly "ziGetValue.vi"("error in"=w181, "Path"="demods/2/sample", "Handle In"=w182) -> ("error out"=w179:errorcluster, "Demod Sample Out"=w183:T1, "Handle Out"=w180:T3)
                    "Demod Sample Out 2" <- w183
                    n44 = Unbundle By Name(w183) -> ("X (Vrms)"=w178:dbl)  [unwired: 2 out]
                  }
                  n45 = Add Array Elements(numeric array=w168) -> (sum=w167:dbl)
                  n46 = Divide(x=w167, y=w165) -> (x/y=w166:dbl)
                  "Imeas (A)" <- w166
                  n47 = Divide(x=w171, y=w166) -> (x/y=w169:dbl)
                  "Resistance (ohm)" <- w169
                }
                frame #4 {
                  n48 = Bundle(w189, w193) -> (w192:cluster{dbl, dbl})  [unwired: 1 in]
                  n49 = Build Array(w189, w193, w185, w196, w191) -> (→"data":dbl[])
                  n50 = Bundle(w189, w188) -> (w190:cluster{dbl, dbl})  [unwired: 1 in]
                  n51 = Build Array (concatenate)(w197, w192) -> (w198:cluster{dbl, "Field Reading":dbl}[])
                  "I vs V" <- w198
                  n52 = Build Array (concatenate)(w186, w190) -> (w187:cluster{dbl, "Field Reading":dbl}[])
                  "R vs V" <- w187
                }
              }
            }
            frame #1 {
              n53 = Wait (ms)(milliseconds to wait=u32 50) -> ()  [unwired: 1 out]
            }
            frame #2 {
              n54 = local read "data"() -> (w201:dbl[])
              n55 = local read "File path"() -> (w203:path)
              n56 = Array To Spreadsheet String(array=w201, 3:"%e" ("format string")) -> (spreadsheet string=w204:string)  [unwired: 1 in]
              n57 = call <vilib>:"Write Characters To File.vi"("append to file? (new file:F)"=TRUE, "character string"=w204, "file path (dialog if empty)"=w203) -> ()  [unwired: 2 in, 1 out]
            }
          }
        }
      }
      n58 = call "ziClose.vi"("Error In"=w43, "Handle In"=w44) -> ()  [unwired: 4 out]
    }
    frame #3 {
      n59 = call "MFLI-Set Value.vi"("Value"=1.0, "Path"="sigouts/0/on", "MFLI Current source/Voltage reader"=w206) -> ()  [unwired: 9 in]
    }
  }
